vi "Test Increment Filename.vi"() -> ()   [LabVIEW 2016]
uses:
  <vilib>/addons/_JKI Toolkits/Caraya/classes/Assert/Assert True.vi
  <vilib>/addons/_JKI Toolkits/Caraya/classes/Assert/Assert.lvclass
  <vilib>/addons/_JKI Toolkits/Caraya/classes/Test/Test.lvclass
panel:
  in  "OK":bool
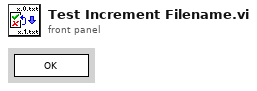
[diagram p1: front panel]
types:
  T1 = enum32{"Invalid", "Standard", "Closed", "Hidden", "Minimized", "Maximized"}
  T2 = enum32{"invalid app kind", "Development System", "Run Time System", "Student Edition", "Embedded LabVIEW", "Evaluation", "Custom"}
  T3 = enum16{"open", "replace", "create", "open or create", "replace or create", "replace or create with confirmation"}
  T4 = cluster{"Core":cluster{"Current VI Reference":refnum<vi>, "Close Panel on Exit?":bool}, "folder path":path}
  T5 = cluster{"Current VI Reference":refnum<vi>, "Close Panel on Exit?":bool}
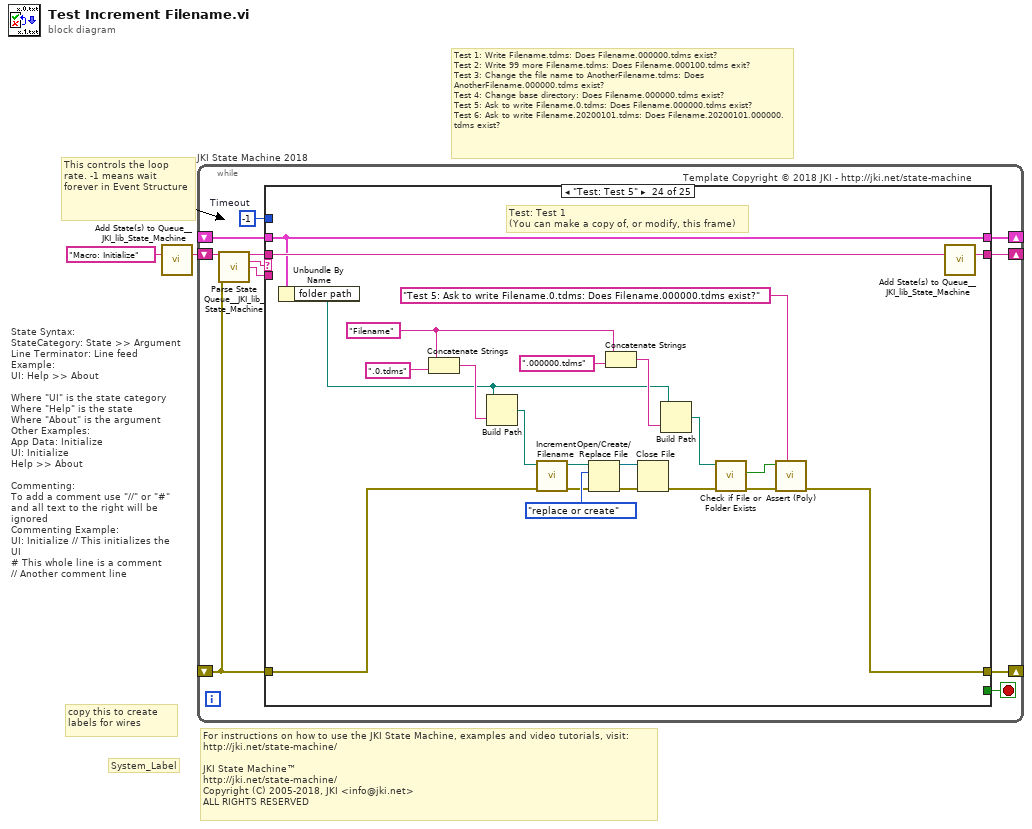
[diagram p0: block diagram]
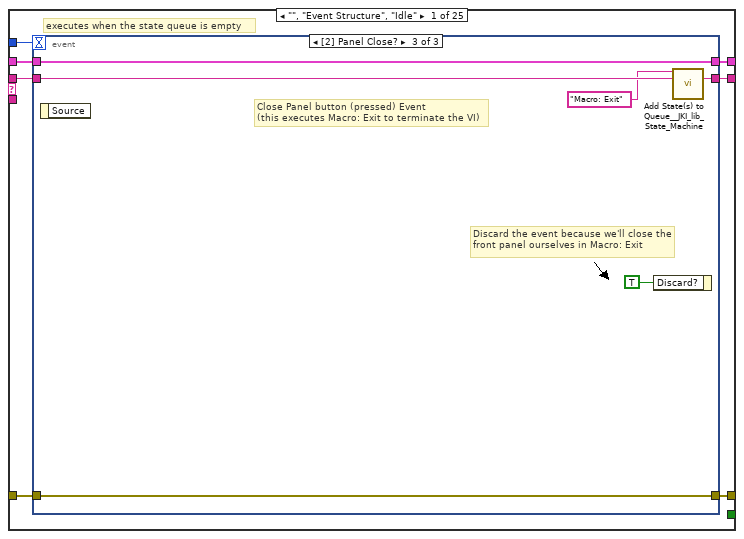
[diagram p2: hidden frame]
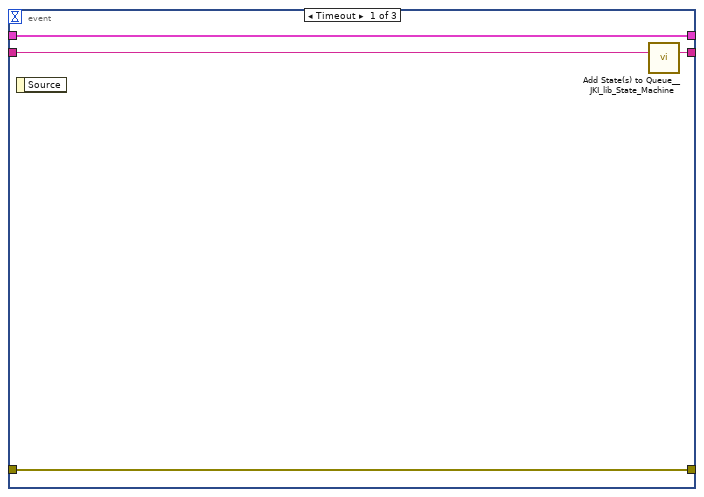
[diagram p3: hidden frame]
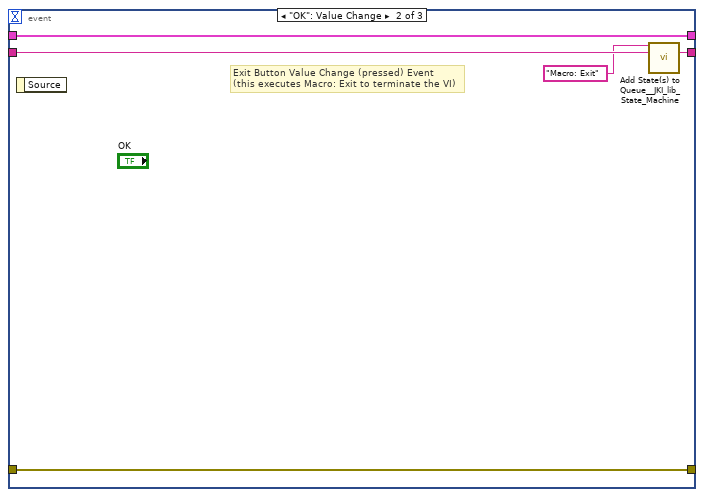
[diagram p4: hidden frame]
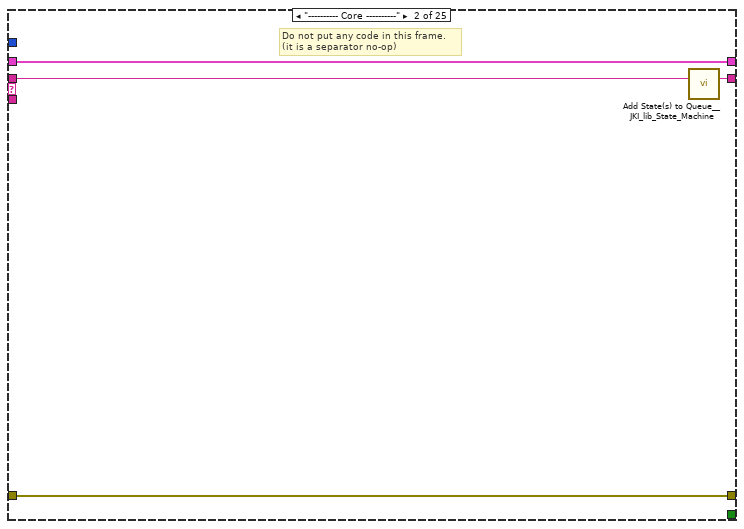
[diagram p5: hidden frame]
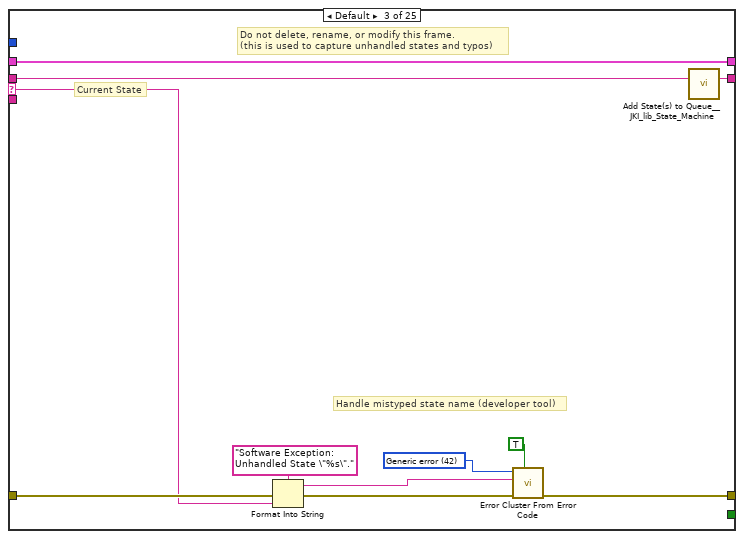
[diagram p6: hidden frame]
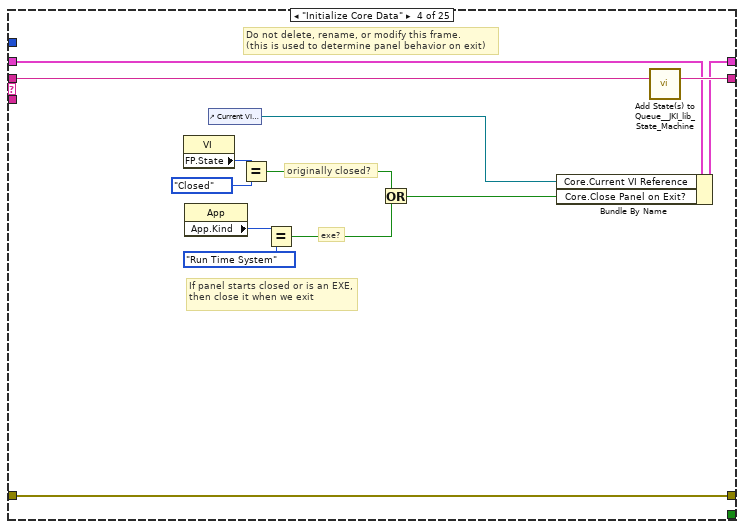
[diagram p7: hidden frame]
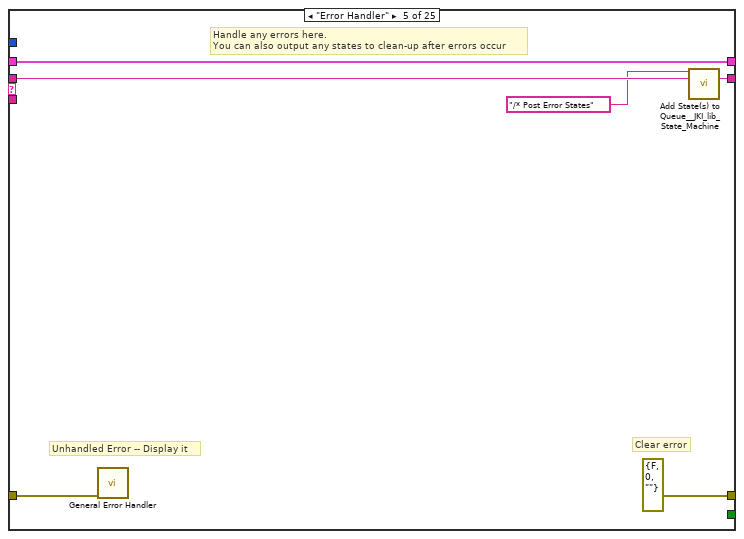
[diagram p8: hidden frame]
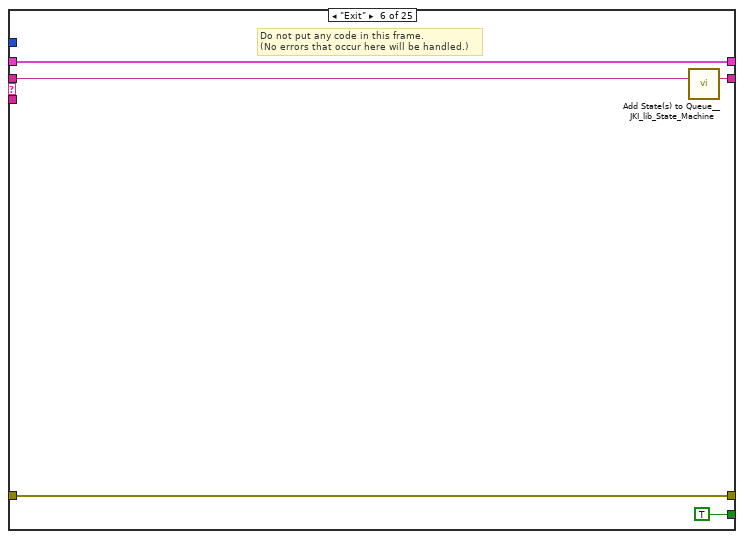
[diagram p9: hidden frame]
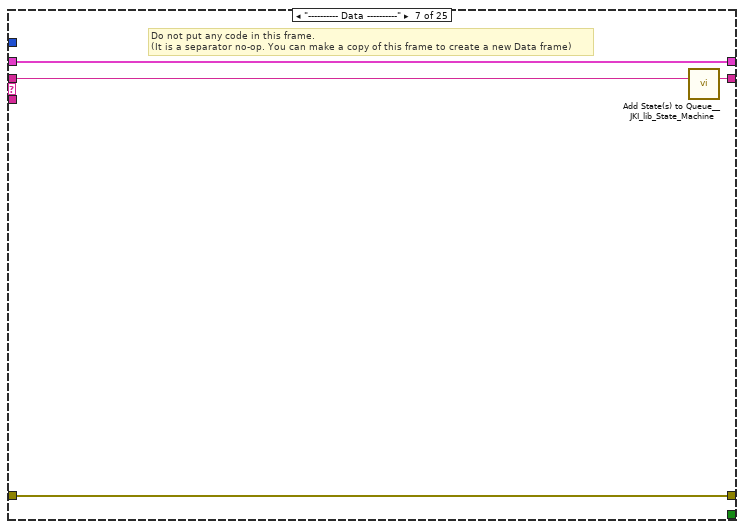
[diagram p10: hidden frame]
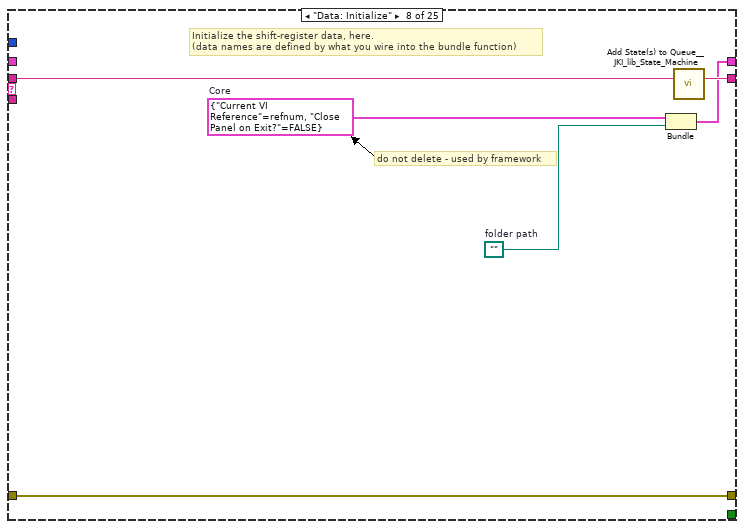
[diagram p11: hidden frame]
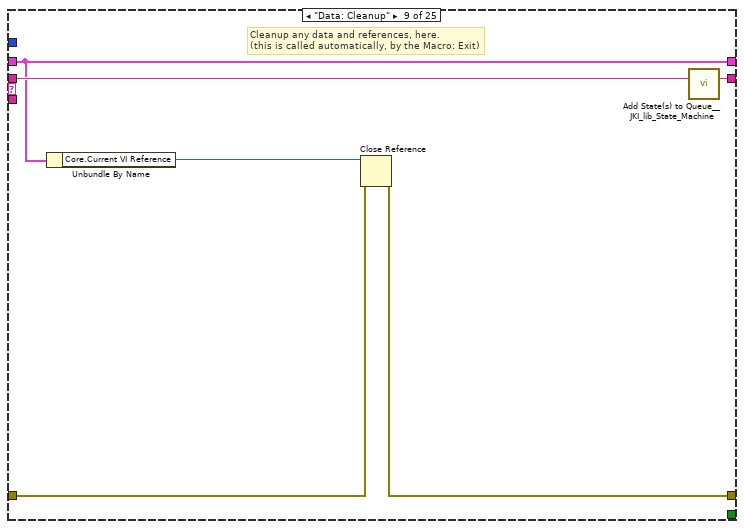
[diagram p12: hidden frame]
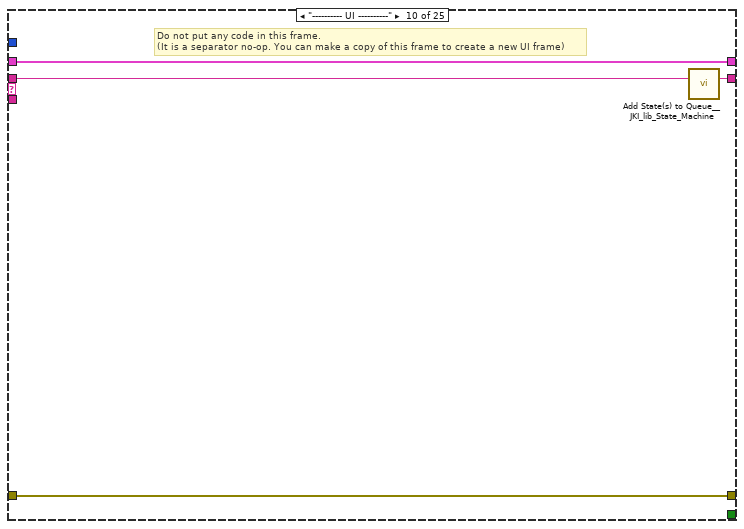
[diagram p13: hidden frame]
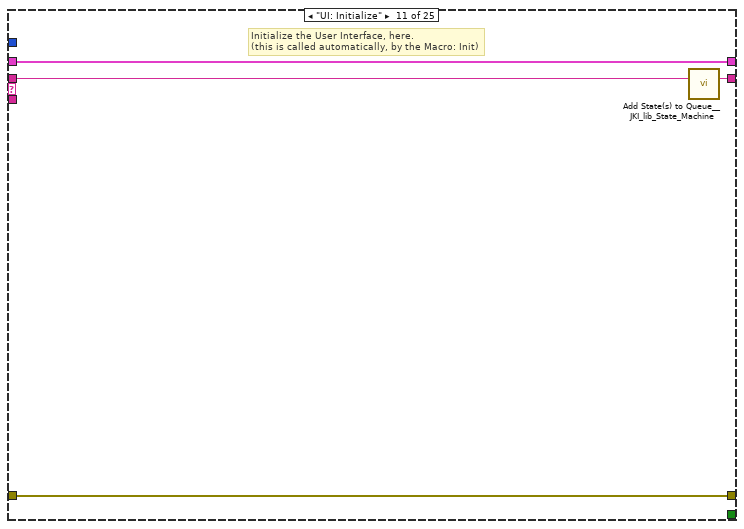
[diagram p14: hidden frame]
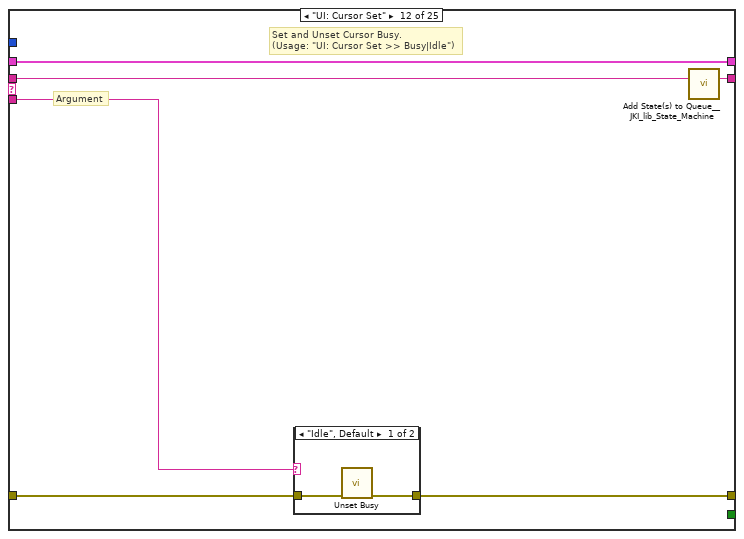
[diagram p15: hidden frame]
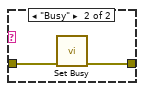
[diagram p16: hidden frame]
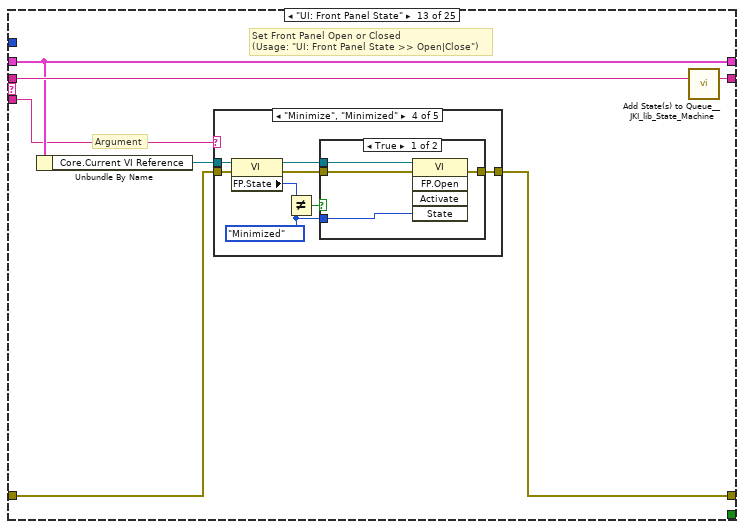
[diagram p17: hidden frame]
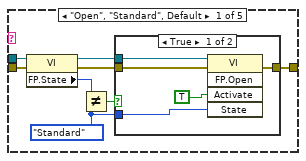
[diagram p18: hidden frame]
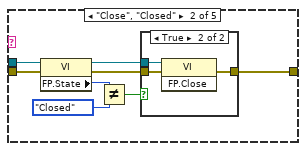
[diagram p20: hidden frame]
diagram:
  # "For instructions on how to use the JKI State Machine, examples and video tutorials, visit:\nhttp://jki.net/state-machine/\n\nJKI State Machine™\nhttp://jki.net/state-machine/\nCopyright (C) 2005-2018, JKI <info@jki.net>\nALL RIGHTS RESERVED"
  # "State Syntax:\nStateCategory: State >> Argument\nLine Terminator: Line feed\nExample:\nUI: Help >> About\n\nWhere \"UI\" is the state category\nWhere \"Help\" is the state\nWhere \"About\" is the argument\nOther Examples:\nApp Data: Initialize\nUI: Initialize\nHelp >> About\n\nCommenting:\nTo add a comment use \"//\" or \"#\" and all text to the right will be ignored\nCommenting Example:\nUI: Initialize // This initializes the UI\n# This whole line is a comment\n// Another comment line"
  # "copy this to create labels for wires"
  # "This controls the loop rate. -1 means wait forever in Event Structure"
  # "System_Label"
  # "Test 1: Write Filename.tdms: Does Filename.000000.tdms exist?\nTest 2: Write 99 more Filename.tdms: Does Filename.000100.tdms exit?\nTest 3: Change the file name to AnotherFilename.tdms: Does AnotherFilename.000000.tdms exist?\nTest 4: Change base directory: Does Filename.000000.tdms exist?\nTest 5: Ask to write Filename.0.tdms: Does Filename.000000.tdms exist?\nTest 6: Ask to write Filename.20200101.tdms: Does Filename.20200101.000000.tdms exist?"
  n1 = call <vilib>:"Add State(s) to Queue__JKI_lib_State_Machine.vi"("State(s) in (\"\")"="Macro: Initialize") -> ("States Out"=w2:string)  [unwired: 14 in]
  n2 = while "JKI State Machine 2018" {
    shift-right: [w6] -> _
    shift-left: _ -> [w5]
    shift-right: [w9] -> _
    shift-left: _ -> [w3]
    shift-right: [w8] -> _
    shift-left: w2 -> [w10]
    stop <- w7 stop-if-true
    w4 = -1  # Timeout
    # "Template Copyright © 2018 JKI - http://jki.net/state-machine"
    n3 = call <vilib>:"Parse State Queue__JKI_lib_State_Machine.vi"("State Queue"=w10, "Error In (no error)"=w3) -> ("Remaining States"=w12:string, "Current State"=w13:string, "Arguments"=w11:string)  [unwired: 11 in]
    n4 = case shown="\"Test: Test 5\"" w13 {
      selector: w13 -> [_ _ w40 _ _ _ _ _ _ _ _ _ _ _ _ _ _ _ _ _ _ _ _ _ _]
      tunnel: w12 -> [w20 w39 w44 w63 w69 w74 w78 w84 w90 w94 w98 w104 w115 w184 w189 w194 w204 w210 w226 w253 w271 w301 w328 w350 w372]
      tunnel: w11 -> [_ _ _ _ _ _ _ _ _ _ _ w99 w109 _ _ _ _ _ _ _ _ _ _ _ _]
      tunnel: w5 -> [w18 w36 w42 w56 w66 w72 w75 _ w85 w91 w96 w102 w111 w181 w186 w191 w201 w206 w214 w233 w254 w280 w309 w330 w352]
      tunnel: [w17 w37 w46 w60 errorcluster {"status"=FALSE, "code"=0, "source"=""} ("error out") w71 w76 w81 w86 w92 w95 w100 w112 w182 w187 w192 w202 w208 w215 w235 w255 w282 w311 w332 w354] -> w9
      tunnel: w3 -> [w16 w37 w45 w60 w65 w71 w76 w81 w87 w92 w95 w101 w113 w182 w187 w192 w202 w208 w216 w236 w256 w283 w303 w333 w355]
      tunnel: [w19 w38 w43 w62 w68 w73 w77 w83 w89 w93 w97 w103 w114 w183 w188 w193 w203 w209 w225 w252 w270 w300 w327 w349 w371] -> w8
      tunnel: [_ _ _ _ _ TRUE _ _ _ _ _ _ _ _ _ _ _ _ _ _ _ _ _ _ _] -> w7
      tunnel: [w15 w36 w42 w61 w66 w72 w75 w82 w85 w91 w96 w102 w111 w181 w186 w191 w201 w207 w213 w233 w254 w280 w309 w330 w352] -> w6
      tunnel: w4 -> [w14 _ _ _ _ _ _ _ _ _ _ _ _ _ _ _ _ _ _ _ _ _ _ _ _]
      frame "", "Event Structure", "Idle" {
        # "executes when the state queue is empty"
        n5 = event shown="[2] Panel Close?" {
          selector: _ -> [_ _ _]
          dyn-events: _ -> [_ _ _]
          timeout: w14 -> [_ _ _]
          tunnel: w20 -> [w24 w29 w35]
          tunnel: [w23 w28 w34] -> w19
          tunnel: w18 -> [w21 w26 w32]
          tunnel: [w22 w27 w33] -> w17
          tunnel: w16 -> [w22 w27 w33]
          tunnel: [w21 w26 w32] -> w15
          event Timeout {
            n6 = event-data() -> ()  [unwired: 1 in, 1 out]
            n7 = call <vilib>:"Add State(s) to Queue__JKI_lib_State_Machine.vi"("State(s) in (\"\")"=w24) -> ("States Out"=w23:string)  [unwired: 14 in]
          }
          event "OK": Value Change {
            # "Exit Button Value Change (pressed) Event\n(this executes Macro: Exit to terminate the VI)"
            n8 = event-data() -> ()  [unwired: 1 in, 1 out]
            n9 = call <vilib>:"Add State(s) to Queue__JKI_lib_State_Machine.vi"("State(s) in Front (\"\")"="Macro: Exit", "State(s) in (\"\")"=w29) -> ("States Out"=w28:string)  [unwired: 13 in]
          }
          event Panel Close? {
            # "Discard the event because we'll close the front panel ourselves in Macro: Exit"
            # "Close Panel button (pressed) Event\n(this executes Macro: Exit to terminate the VI)"
            n10 = event-data() -> ()  [unwired: 1 in, 1 out]
            n11 = event-data ("Event Filter Node")("Discard?"=TRUE) -> ()  [unwired: 1 in, 1 out]
            n12 = call <vilib>:"Add State(s) to Queue__JKI_lib_State_Machine.vi"("State(s) in Front (\"\")"="Macro: Exit", "State(s) in (\"\")"=w35) -> ("States Out"=w34:string)  [unwired: 13 in]
          }
        }
      }
      frame "---------- Core ----------" {
        # "Do not put any code in this frame.\n(it is a separator no-op)"
        n13 = call <vilib>:"Add State(s) to Queue__JKI_lib_State_Machine.vi"("State(s) in (\"\")"=w39) -> ("States Out"=w38:string)  [unwired: 14 in]
      }
      frame Default {
        w49 = 42 items=["No error", "Argument error", "Memory is full", "Out of zone", "End of file", "File already open", "Generic file I/O error", "File not found", "File permission error", "Disk is full", "Duplicate path", "Too many files open", "System feature not enabled", "Resource file not found", "Cannot add resource", "Resource not found", "Image not found", "Image memory error", "Pen does not exist", "Config type invalid", "Config token not found", "Config parse error", "Config memory error", "Bad external code format", "Bad external code offset", "External code not present", "Null window", "Destroy window error", "Null menu", "Print aborted", "Bad print record", "Print driver error", "Windows error during printing", "Memory error during printing", "Print dialog error", "Generic print error", "Invalid device refnum", "Device not found", "Device parameter error", "Device unit error", "Cannot open device", "Device call aborted", "Generic error", "Cancelled by user", "Object ID too low", "Object ID too high", "Object not in heap", "Unknown heap", "Unknown object (invalid DefProc)", "Unknown object (DefProc not in table)", "Message out of range", "Invalid (null) method", "Unknown message", "Manager call not supported", "Bad address", "Network operation in progress", "Network operation timed out", "Connection is busy", "Network attribute not supported", "Network error", "Address in use", "System out of memory", "Connection aborted", "Connection refused", "Not connected", "Already connected", "Connection closed", "Initialization error (interapplication manager)", "Bad occurrence", "Wait on unbound occurrence handler", "Occurrence queue overflow", "Datalog type conflict", "Unused", "Unrecognized type (interapplication manager)", "Memory corrupt", "Failed to make temporary DLL", "Old CIN version", "Drag socket not found", "Failed to load drop-object", "Failed to register OLE object", "Failed to release OLE object", "Format specifier type mismatch", "Unknown format specifier", "Too few format specifiers", "Too many format specifiers", "Scan failed", "Newer CIN version", "Error converting to variant", "Runtime menu error", "Password tampered", "Variant attribute not found", "Incompatible variant data type", "Event data is not available", "Event Store is not present", "Occurrence is not found", "Event Queue is not created", "Event info is not available", "Refnum passed is NULL", "Error retrieving Class GUID", "Error retrieving CoClass GUID", "Error retrieving TypeLib GUID.", "Bad built application magic bytes.", "Specific driver is different from the specific driver associated with the Logical Name.", "There is no session opened to the class driver.", "Max Error", "MAX - Error with config objects", "MAX - Error loading configuration", "MAX - Group not supported"]
        # "Current State"
        # "Do not delete, rename, or modify this frame.\n(this is used to capture unhandled states and typos)"
        # "Handle mistyped state name (developer tool)"
        n14 = Format Into String(format string="Software Exception: Unhandled State \"%s\"." ("message"), error in=w45, w40) -> (resulting string=w48:string, error out=w47:errorcluster)  [unwired: 1 in]
        n15 = call <vilib>:"Error Cluster From Error Code.vi"("show call chain? (False)"=TRUE, "error in (no error)"=w47, "error message (\"\")"=w48, "error code (0)"=w49) -> ("error out"=w46:errorcluster)  [unwired: 5 in]
        n16 = call <vilib>:"Add State(s) to Queue__JKI_lib_State_Machine.vi"("State(s) in (\"\")"=w44) -> ("States Out"=w43:string)  [unwired: 14 in]
      }
      frame "Initialize Core Data" {
        # "Do not delete, rename, or modify this frame.\n(this is used to determine panel behavior on exit)"
        # "originally closed?"
        # "exe?"
        # "If panel starts closed or is an EXE, then close it when we exit"
        n17 = property on="Property Node" class="VI"() -> ("FP.State"=w53:T1)  [unwired: 2 in, 2 out]
        n18 = property on="Property Node" class="App"() -> ("App.Kind"=w59:T2)  [unwired: 2 in, 2 out]
        n19 = control-ref of="Current VI Reference"() -> (w54:refnum<vi>)
        n20 = Equal?(x=w53, y=T1."Closed" ("Front Panel Window:State")) -> (x = y?=w51:bool)
        n21 = Equal?(x=w59, y=T2."Run Time System" ("Application:Kind")) -> (x = y?=w57:bool)
        n22 = Or(x=w51, y=w57) -> (x .or. y?=w55:bool)
        n23 = Bundle By Name(cluster=w56, "Core.Current VI Reference"=w54, "Core.Close Panel on Exit?"=w55) -> (w61:T4)
        n24 = call <vilib>:"Add State(s) to Queue__JKI_lib_State_Machine.vi"("State(s) in (\"\")"=w63) -> ("States Out"=w62:string)  [unwired: 14 in]
      }
      frame "Error Handler" {
        # "Unhandled Error -- Display it"
        # "Handle any errors here.\nYou can also output any states to clean-up after errors occur"
        # "Clear error"
        n25 = call <vilib>:"General Error Handler.vi"("error in (no error)"=w65) -> ()  [unwired: 10 in, 5 out]
        n26 = call <vilib>:"Add State(s) to Queue__JKI_lib_State_Machine.vi"("State(s) in Front (\"\")"="/* Post Error States", "State(s) in (\"\")"=w69) -> ("States Out"=w68:string)  [unwired: 13 in]
      }
      frame "Exit" {
        # "Do not put any code in this frame.\n(No errors that occur here will be handled.)"
        n27 = call <vilib>:"Add State(s) to Queue__JKI_lib_State_Machine.vi"("State(s) in (\"\")"=w74) -> ("States Out"=w73:string)  [unwired: 14 in]
      }
      frame "---------- Data ----------" {
        # "Do not put any code in this frame.\n(It is a separator no-op. You can make a copy of this frame to create a new Data frame)"
        n28 = call <vilib>:"Add State(s) to Queue__JKI_lib_State_Machine.vi"("State(s) in (\"\")"=w78) -> ("States Out"=w77:string)  [unwired: 14 in]
      }
      frame "Data: Initialize" {
        w79 = path ""  # folder path
        w80 = T5 {"Current VI Reference"=refnum, "Close Panel on Exit?"=FALSE}  # Core
        # "do not delete - used by framework"
        # "Initialize the shift-register data, here.\n(data names are defined by what you wire into the bundle function)"
        n29 = Bundle("Core"=w80, "folder path"=w79) -> (w82:T4)  [unwired: 1 in]
        n30 = call <vilib>:"Add State(s) to Queue__JKI_lib_State_Machine.vi"("State(s) in (\"\")"=w84) -> ("States Out"=w83:string)  [unwired: 14 in]
      }
      frame "Data: Cleanup" {
        # "Cleanup any data and references, here.\n(this is called automatically, by the Macro: Exit)"
        n31 = Unbundle By Name(w85) -> ("Core.Current VI Reference"=w88:refnum<vi>)
        n32 = Close Reference(reference=w88, error in (no error)=w87) -> (error out=w86:errorcluster)
        n33 = call <vilib>:"Add State(s) to Queue__JKI_lib_State_Machine.vi"("State(s) in (\"\")"=w90) -> ("States Out"=w89:string)  [unwired: 14 in]
      }
      frame "---------- UI ----------" {
        # "Do not put any code in this frame.\n(It is a separator no-op. You can make a copy of this frame to create a new UI frame)"
        n34 = call <vilib>:"Add State(s) to Queue__JKI_lib_State_Machine.vi"("State(s) in (\"\")"=w94) -> ("States Out"=w93:string)  [unwired: 14 in]
      }
      frame "UI: Initialize" {
        # "Initialize the User Interface, here.\n(this is called automatically, by the Macro: Init)"
        n35 = call <vilib>:"Add State(s) to Queue__JKI_lib_State_Machine.vi"("State(s) in (\"\")"=w98) -> ("States Out"=w97:string)  [unwired: 14 in]
      }
      frame "UI: Cursor Set" {
        # "Argument"
        # "Set and Unset Cursor Busy.\n(Usage: \"UI: Cursor Set >> Busy|Idle\")"
        n36 = case shown="\"Idle\", Default" w99 {
          tunnel: w101 -> [w106 w108]
          tunnel: [w105 w107] -> w100
          frame "Idle", Default {
            n37 = call <vilib>:"Unset Busy.vi"("error in (no error)"=w106) -> ("error out"=w105:errorcluster)  [unwired: 10 in]
          }
          frame "Busy" {
            n38 = call <vilib>:"Set Busy.vi"("error in (no error)"=w108) -> ("error out"=w107:errorcluster)  [unwired: 9 in, 1 out]
          }
        }
        n39 = call <vilib>:"Add State(s) to Queue__JKI_lib_State_Machine.vi"("State(s) in (\"\")"=w104) -> ("States Out"=w103:string)  [unwired: 14 in]
      }
      frame "UI: Front Panel State" {
        # "Argument"
        # "Set Front Panel Open or Closed\n(Usage: \"UI: Front Panel State >> Open|Close\")"
        n40 = Unbundle By Name(w111) -> ("Core.Current VI Reference"=w110:refnum<vi>)
        n41 = case shown="\"Minimize\", \"Minimized\"" w109 {
          tunnel: w113 -> [w121 w136 w147 w160 w173]
          tunnel: [w123 w137 w149 w162 w175] -> w112
          tunnel: w110 -> [w122 w134 w148 w161 w174]
          frame "Open", "Standard", Default {
            w116 = T1."Standard" ("State")
            n42 = property on="Property Node" class="VI"(reference=w122, error in=w121) -> (reference out=w119:refnum<vi>, error out=w120:errorcluster, "FP.State"=w118:T1)
            n43 = Not Equal?(x=w118, y=w116) -> (x != y?=w117:bool)
            n44 = case shown="True" w117 {
              tunnel: [w127 w129] -> w123
              tunnel: w120 -> [w126 w129]
              tunnel: w119 -> [w125 _]
              tunnel: w116 -> [w124 _]
              frame True {
                n45 = invoke on="Invoke Node" class="VI" method="FP.Open"(reference=w125, error in=w126, "Activate"=TRUE, "State"=w124) -> (error out=w127:errorcluster)  [unwired: 1 in, 4 out]
              }
              frame False {
              }
            }
          }
          frame "Close", "Closed" {
            n46 = property on="Property Node" class="VI"(reference=w134, error in=w136) -> (reference out=w133:refnum<vi>, error out=w135:errorcluster, "FP.State"=w131:T1)
            n47 = Not Equal?(x=w131, y=T1."Closed" ("Front Panel Window:State")) -> (x != y?=w130:bool)
            n48 = case shown="True" w130 {
              tunnel: [w138 w141] -> w137
              tunnel: w135 -> [w138 w140]
              tunnel: w133 -> [_ w139]
              frame False {
              }
              frame True {
                n49 = invoke on="Invoke Node" class="VI" method="FP.Close"(reference=w139, error in=w140) -> (error out=w141:errorcluster)  [unwired: 1 in, 2 out]
              }
            }
          }
          frame "Hidden", "Hide" {
            w142 = T1."Hidden" ("State")
            n50 = property on="Property Node" class="VI"(reference=w148, error in=w147) -> (reference out=w145:refnum<vi>, error out=w146:errorcluster, "FP.State"=w144:T1)
            n51 = Not Equal?(x=w144, y=w142) -> (x != y?=w143:bool)
            n52 = case shown="True" w143 {
              tunnel: [w153 w154] -> w149
              tunnel: w146 -> [w152 w154]
              tunnel: w145 -> [w151 _]
              tunnel: w142 -> [w150 _]
              frame True {
                n53 = invoke on="Invoke Node" class="VI" method="FP.Open"(reference=w151, error in=w152, "State"=w150) -> (error out=w153:errorcluster)  [unwired: 2 in, 4 out]
              }
              frame False {
              }
            }
          }
          frame "Minimize", "Minimized" {
            w155 = T1."Minimized" ("State")
            n54 = property on="Property Node" class="VI"(reference=w161, error in=w160) -> (reference out=w158:refnum<vi>, error out=w159:errorcluster, "FP.State"=w157:T1)
            n55 = Not Equal?(x=w157, y=w155) -> (x != y?=w156:bool)
            n56 = case shown="True" w156 {
              tunnel: [w166 w167] -> w162
              tunnel: w159 -> [w165 w167]
              tunnel: w158 -> [w164 _]
              tunnel: w155 -> [w163 _]
              frame True {
                n57 = invoke on="Invoke Node" class="VI" method="FP.Open"(reference=w164, error in=w165, "State"=w163) -> (error out=w166:errorcluster)  [unwired: 2 in, 4 out]
              }
              frame False {
              }
            }
          }
          frame "Maximize", "Maximized" {
            w168 = T1."Maximized" ("State")
            n58 = property on="Property Node" class="VI"(reference=w174, error in=w173) -> (reference out=w171:refnum<vi>, error out=w172:errorcluster, "FP.State"=w170:T1)
            n59 = Not Equal?(x=w170, y=w168) -> (x != y?=w169:bool)
            n60 = case shown="True" w169 {
              tunnel: [w179 w180] -> w175
              tunnel: w172 -> [w178 w180]
              tunnel: w171 -> [w177 _]
              tunnel: w168 -> [w176 _]
              frame True {
                n61 = invoke on="Invoke Node" class="VI" method="FP.Open"(reference=w177, error in=w178, "State"=w176) -> (error out=w179:errorcluster)  [unwired: 2 in, 4 out]
              }
              frame False {
              }
            }
          }
        }
        n62 = call <vilib>:"Add State(s) to Queue__JKI_lib_State_Machine.vi"("State(s) in (\"\")"=w115) -> ("States Out"=w114:string)  [unwired: 14 in]
      }
      frame "---------- Macro ----------" {
        # "Do not put any code in this frame.\n(It is a separator no-op. You can make a copy of this frame to create a new Macro frame)"
        n63 = call <vilib>:"Add State(s) to Queue__JKI_lib_State_Machine.vi"("State(s) in (\"\")"=w184) -> ("States Out"=w183:string)  [unwired: 14 in]
      }
      frame "Macro: Initialize" {
        w185 = "Data: Initialize\nInitialize Core Data\nUI: Initialize\nUI: Front Panel State >> Open\nMacro: Tests\nMacro: Exit"  # Data: Initialize Initialize Core Data UI: Initialize UI: Front Panel State >> Open Macro: Tests Macro: Exit
        # "Initialization Macro\n(This is called once, when the VI starts)"
        n64 = call <vilib>:"Add State(s) to Queue__JKI_lib_State_Machine.vi"("State(s) in Front (\"\")"=w185, "State(s) in (\"\")"=w189) -> ("States Out"=w188:string)  [unwired: 13 in]
      }
      frame "Macro: Tests" {
        # "Do not put any code in this frame.\n(It is a separator no-op. You can make a copy of this frame to create a new Macro frame)"
        n65 = call <vilib>:"Add State(s) to Queue__JKI_lib_State_Machine.vi"("State(s) in Front (\"\")"="Test: Initialize\nTest: Test 1\nTest: Test 2\nTest: Test 3\nTest: Test 4\nTest: Test 5\nTest: Test 6" ("State(s) in Front (\"\")"), "State(s) in (\"\")"=w194) -> ("States Out"=w193:string)  [unwired: 13 in]
      }
      frame "Macro: Exit" {
        # "Exit Macro\n(This is called once, when the VI exits)"
        n66 = Unbundle By Name(w201) -> ("Core.Close Panel on Exit?"=w200:bool)
        n67 = Select(t="UI: Front Panel State >> Close", s=w200, f="") -> (s? t:f=w197:string)
        n68 = call <vilib>:"Add State(s) to Queue__JKI_lib_State_Machine.vi"("State(s) in (\"\")"=w197, "State(s) at Back (\"\")"="Data: Cleanup\nExit") -> ("States Out"=w195:string)  [unwired: 13 in]
        n69 = call <vilib>:"Add State(s) to Queue__JKI_lib_State_Machine.vi"("State(s) in Front (\"\")"=w195, "State(s) in (\"\")"=w204) -> ("States Out"=w203:string)  [unwired: 13 in]
      }
      frame "---------- Test ----------" {
        # "Test\n(You can make a copy of, or modify, this frame)"
        n70 = Unbundle By Name(w206) -> ("folder path"=w205:path)
        n71 = Bundle By Name(cluster=w206, "folder path"=w205) -> (w207:T4)
        n72 = call <vilib>:"Add State(s) to Queue__JKI_lib_State_Machine.vi"("State(s) in (\"\")"=w210) -> ("States Out"=w209:string)  [unwired: 14 in]
      }
      frame "Test: Initialize" {
        # "Test: Initialize.\n(You can make a copy of, or modify, this frame)"
        n73 = call <userlib>:"Temporary Directory__ogtk.vi"("Relative path (.)"=path "File Utilities") -> ("Temporary Directory (+ Relative)"=w212:path)
        n74 = call <vilib>:"Define Test.vi"("error in (no error)"=w216) -> ("error out"=w224:errorcluster)  [unwired: 10 in]
        n75 = call <vilib>:"Check if File or Folder Exists.vi"("error in (no error)"=w224, "path"=w212) -> ("error out"=w220:errorcluster, "file or folder exists?"=w218:bool, "dup path"=w219:path)  [unwired: 7 in]
        n76 = case shown="True" w218 {
          tunnel: w219 -> [_ w229]
          tunnel: w220 -> [w227 w231]
          tunnel: [w227 w230] -> w223
          frame False {
          }
          frame True {
            n77 = call <userlib>:"Delete Recursive__ogtk.vi"("error in (no error)"=w231, "Recursive? (FALSE)"=TRUE, "Path"=w229) -> ("error out"=w230:errorcluster)  [unwired: 7 in, 1 out]
          }
        }
        n78 = Build Path(base path=w212, name or relative path="Folder 1") -> (appended path=w222:path)
        n79 = call <userlib>:"Create Dir if Non-Existant__ogtk.vi"("error in (no error)"=w223, "Directory Path"=w222) -> ("error out"=w215:errorcluster, "dup Directory Path"=w211:path)  [unwired: 7 in, 1 out]
        n80 = Bundle By Name(cluster=w214, "folder path"=w211) -> (w213:T4)
        n81 = call <vilib>:"Add State(s) to Queue__JKI_lib_State_Machine.vi"("State(s) in (\"\")"=w226) -> ("States Out"=w225:string)  [unwired: 14 in]
      }
      frame "Test: Test 1" {
        w250 = "Filename" ("name or relative path")
        # "Test: Test 1\n(You can make a copy of, or modify, this frame)"
        n82 = Unbundle By Name(w233) -> ("folder path"=w234:path)
        n83 = Concatenate Strings(w250, ".tdms" ("name or relative path")) -> (w251:string)
        n84 = Build Path(base path=w234, name or relative path=w251) -> (appended path=w239:path)
        n85 = call "Increment Filename.vi"("error in (no error)"=w236, "path"=w239) -> ("error out"=w241:errorcluster, "modified path"=w240:path)  [unwired: 8 in]
        n86 = Open/Create/Replace File(file path (use dialog)=w240, error in=w241, operation (0:open)=T3."replace or create") -> (refnum out=w238:refnum<file>, error out=w237:errorcluster)  [unwired: 3 in, 1 out]
        n87 = Concatenate Strings(w250, ".000000.tdms" ("name or relative path")) -> (w249:string)
        n88 = Close File(refnum=w238, error in=w237) -> (error out=w243:errorcluster)  [unwired: 1 out]
        n89 = Build Path(base path=w234, name or relative path=w249) -> (appended path=w244:path)
        n90 = call <vilib>:"Check if File or Folder Exists.vi"("error in (no error)"=w243, "path"=w244) -> ("error out"=w245:errorcluster, "file or folder exists?"=w246:bool)  [unwired: 7 in, 1 out]
        n91 = call-poly <vilib>:"Assert (Poly).vi"("Label"="Test 1: Write Filename.tdms: Does Filename.000000.tdms exist?", "error in (no error)"=w245, "True?"=w246) -> ("error out"=w235:errorcluster)  [unwired: 8 in]
        n92 = call <vilib>:"Add State(s) to Queue__JKI_lib_State_Machine.vi"("State(s) in (\"\")"=w253) -> ("States Out"=w252:string)  [unwired: 14 in]
      }
      frame "Test: Test 2" {
        w258 = "Filename" ("name or relative path")
        # "Test: Test 2\n(You can make a copy of, or modify, this frame)"
        n93 = Unbundle By Name(w254) -> ("folder path"=w257:path)
        n94 = Concatenate Strings(w258, ".tdms" ("name or relative path")) -> (w268:string)
        n95 = Build Path(base path=w257, name or relative path=w268) -> (appended path=w262:path)
        n96 = for {
          N: 100 -> [_]
          tunnel: w262 -> [w274]
          shift-right: [w278] -> w261
          shift-left: w256 -> [w279]
          n97 = call "Increment Filename.vi"("error in (no error)"=w279, "path"=w274) -> ("error out"=w276:errorcluster, "modified path"=w275:path)  [unwired: 8 in]
          n98 = Open/Create/Replace File(file path (use dialog)=w275, error in=w276, operation (0:open)=T3."replace or create") -> (refnum out=w273:refnum<file>, error out=w272:errorcluster)  [unwired: 3 in, 1 out]
          n99 = Close File(refnum=w273, error in=w272) -> (error out=w278:errorcluster)  [unwired: 1 out]
        }
        n100 = Concatenate Strings(w258, ".000100.tdms" ("name or relative path")) -> (w267:string)
        n101 = Build Path(base path=w257, name or relative path=w267) -> (appended path=w260:path)
        n102 = call <vilib>:"Check if File or Folder Exists.vi"("error in (no error)"=w261, "path"=w260) -> ("error out"=w264:errorcluster, "file or folder exists?"=w259:bool)  [unwired: 7 in, 1 out]
        n103 = call-poly <vilib>:"Assert (Poly).vi"("Label"="Test 2: Write 100 more Filename.tdms: Does Filename.000100.tdms exit?", "error in (no error)"=w264, "True?"=w259) -> ("error out"=w255:errorcluster)  [unwired: 8 in]
        n104 = call <vilib>:"Add State(s) to Queue__JKI_lib_State_Machine.vi"("State(s) in (\"\")"=w271) -> ("States Out"=w270:string)  [unwired: 14 in]
      }
      frame "Test: Test 3" {
        w284 = "AnotherFilename" ("name or relative path")
        # "Test: Test 3\n(You can make a copy of, or modify, this frame)"
        n105 = Unbundle By Name(w280) -> ("folder path"=w281:path)
        n106 = Concatenate Strings(w284, ".tdms" ("name or relative path")) -> (w286:string)
        n107 = Build Path(base path=w281, name or relative path=w286) -> (appended path=w291:path)
        n108 = call "Increment Filename.vi"("error in (no error)"=w283, "path"=w291) -> ("error out"=w293:errorcluster, "modified path"=w292:path)  [unwired: 8 in]
        n109 = Concatenate Strings(w284, ".000000.tdms" ("name or relative path")) -> (w285:string)
        n110 = Open/Create/Replace File(file path (use dialog)=w292, error in=w293, operation (0:open)=T3."replace or create") -> (refnum out=w290:refnum<file>, error out=w289:errorcluster)  [unwired: 3 in, 1 out]
        n111 = Close File(refnum=w290, error in=w289) -> (error out=w295:errorcluster)  [unwired: 1 out]
        n112 = Build Path(base path=w281, name or relative path=w285) -> (appended path=w296:path)
        n113 = call <vilib>:"Check if File or Folder Exists.vi"("error in (no error)"=w295, "path"=w296) -> ("error out"=w297:errorcluster, "file or folder exists?"=w298:bool)  [unwired: 7 in, 1 out]
        n114 = call-poly <vilib>:"Assert (Poly).vi"("Label"="Test 3: Change the file name to AnotherFilename.tdms: Does AnotherFilename.000000.tdms exist?", "error in (no error)"=w297, "True?"=w298) -> ("error out"=w282:errorcluster)  [unwired: 8 in]
        n115 = call <vilib>:"Add State(s) to Queue__JKI_lib_State_Machine.vi"("State(s) in (\"\")"=w301) -> ("States Out"=w300:string)  [unwired: 14 in]
      }
      frame "Test: Test 4" {
        w310 = "Filename" ("name or relative path")
        # "Test: test 4\n(You can make a copy of, or modify, this frame)"
        n116 = Unbundle By Name(w309) -> ("folder path"=w308:path)
        n117 = Strip Path(path=w308) -> (stripped path=w306:path)  [unwired: 1 out]
        n118 = Build Path(base path=w306, name or relative path="Folder 2") -> (appended path=w304:path)
        n119 = Concatenate Strings(w310, ".tdms" ("name or relative path")) -> (w313:string)
        n120 = call <userlib>:"Create Dir if Non-Existant__ogtk.vi"("error in (no error)"=w303, "Directory Path"=w304) -> ("error out"=w302:errorcluster, "dup Directory Path"=w305:path)  [unwired: 7 in, 1 out]
        n121 = Build Path(base path=w305, name or relative path=w313) -> (appended path=w323:path)
        n122 = call "Increment Filename.vi"("error in (no error)"=w302, "path"=w323) -> ("error out"=w321:errorcluster, "modified path"=w322:path)  [unwired: 8 in]
        n123 = Open/Create/Replace File(file path (use dialog)=w322, error in=w321, operation (0:open)=T3."replace or create") -> (refnum out=w324:refnum<file>, error out=w325:errorcluster)  [unwired: 3 in, 1 out]
        n124 = Concatenate Strings(w310, ".000000.tdms" ("name or relative path")) -> (w312:string)
        n125 = Close File(refnum=w324, error in=w325) -> (error out=w319:errorcluster)  [unwired: 1 out]
        n126 = Build Path(base path=w305, name or relative path=w312) -> (appended path=w318:path)
        n127 = call <vilib>:"Check if File or Folder Exists.vi"("error in (no error)"=w319, "path"=w318) -> ("error out"=w317:errorcluster, "file or folder exists?"=w316:bool)  [unwired: 7 in, 1 out]
        n128 = call-poly <vilib>:"Assert (Poly).vi"("Label"="Test 4: Change base directory: Does Filename.000000.tdms exist?", "error in (no error)"=w317, "True?"=w316) -> ("error out"=w311:errorcluster)  [unwired: 8 in]
        n129 = call <vilib>:"Add State(s) to Queue__JKI_lib_State_Machine.vi"("State(s) in (\"\")"=w328) -> ("States Out"=w327:string)  [unwired: 14 in]
      }
      frame "Test: Test 5" {
        w347 = "Filename" ("name or relative path")
        # "Test: Test 1\n(You can make a copy of, or modify, this frame)"
        n130 = Unbundle By Name(w330) -> ("folder path"=w331:path)
        n131 = Concatenate Strings(w347, ".0.tdms" ("name or relative path")) -> (w348:string)
        n132 = Build Path(base path=w331, name or relative path=w348) -> (appended path=w336:path)
        n133 = call "Increment Filename.vi"("error in (no error)"=w333, "path"=w336) -> ("error out"=w338:errorcluster, "modified path"=w337:path)  [unwired: 8 in]
        n134 = Open/Create/Replace File(file path (use dialog)=w337, error in=w338, operation (0:open)=T3."replace or create") -> (refnum out=w335:refnum<file>, error out=w334:errorcluster)  [unwired: 3 in, 1 out]
        n135 = Concatenate Strings(w347, ".000000.tdms" ("name or relative path")) -> (w346:string)
        n136 = Close File(refnum=w335, error in=w334) -> (error out=w340:errorcluster)  [unwired: 1 out]
        n137 = Build Path(base path=w331, name or relative path=w346) -> (appended path=w341:path)
        n138 = call <vilib>:"Check if File or Folder Exists.vi"("error in (no error)"=w340, "path"=w341) -> ("error out"=w342:errorcluster, "file or folder exists?"=w343:bool)  [unwired: 7 in, 1 out]
        n139 = call-poly <vilib>:"Assert (Poly).vi"("Label"="Test 5: Ask to write Filename.0.tdms: Does Filename.000000.tdms exist?", "error in (no error)"=w342, "True?"=w343) -> ("error out"=w332:errorcluster)  [unwired: 8 in]
        n140 = call <vilib>:"Add State(s) to Queue__JKI_lib_State_Machine.vi"("State(s) in (\"\")"=w350) -> ("States Out"=w349:string)  [unwired: 14 in]
      }
      frame "Test: Test 6" {
        w369 = "Filename.20200101" ("name or relative path")
        # "Test: Test 1\n(You can make a copy of, or modify, this frame)"
        n141 = Unbundle By Name(w352) -> ("folder path"=w353:path)
        n142 = Concatenate Strings(w369, ".tdms" ("name or relative path")) -> (w370:string)
        n143 = Build Path(base path=w353, name or relative path=w370) -> (appended path=w358:path)
        n144 = call "Increment Filename.vi"("error in (no error)"=w355, "path"=w358) -> ("error out"=w360:errorcluster, "modified path"=w359:path)  [unwired: 8 in]
        n145 = Open/Create/Replace File(file path (use dialog)=w359, error in=w360, operation (0:open)=T3."replace or create") -> (refnum out=w357:refnum<file>, error out=w356:errorcluster)  [unwired: 3 in, 1 out]
        n146 = Concatenate Strings(w369, ".000000.tdms" ("name or relative path")) -> (w368:string)
        n147 = Close File(refnum=w357, error in=w356) -> (error out=w362:errorcluster)  [unwired: 1 out]
        n148 = Build Path(base path=w353, name or relative path=w368) -> (appended path=w363:path)
        n149 = call <vilib>:"Check if File or Folder Exists.vi"("error in (no error)"=w362, "path"=w363) -> ("error out"=w364:errorcluster, "file or folder exists?"=w365:bool)  [unwired: 7 in, 1 out]
        n150 = call-poly <vilib>:"Assert (Poly).vi"("Label"="Test 6: Ask to write Filename.20200101.tdms: Does Filename.20200101.000000.tdms exist?", "error in (no error)"=w364, "True?"=w365) -> ("error out"=w354:errorcluster)  [unwired: 8 in]
        n151 = call <vilib>:"Add State(s) to Queue__JKI_lib_State_Machine.vi"("State(s) in (\"\")"=w372) -> ("States Out"=w371:string)  [unwired: 14 in]
      }
    }
  }
